vi "NewTemplate.GetBroadcasts.vi"(11 "NewTemplate in":refnum<class "Header.lvclass">) -> (2 "TemplateModule":cluster{"Broadcasts":T1, "Broadcasts":T2}, 3 "NewTemplate out":refnum<class "Header.lvclass">)   [LabVIEW 2024, in "Header.lvclass"]
uses:
  Header.lvclass
  JQMHCore/Module/StandardBroadcasts.ctl
  JQMHCore/Shared/Died.ctl
  JQMHCore/Module/Started.ctl
  Broadcast Events--cluster.ctl
  Stopped.ctl
  JQMHCore/Module/RQMHModule.lvclass/RQMHModule.ctl
  Header.lvclass/Header.ctl
  JQMHCore/Module/RQMHModule.lvclass
  C:/DevOps/CORTEX/JQMH/JQMHCore/Module/RQMHModule.lvclass
  C:/DevOps/CORTEX/JQMH/ModuleTemplates/Header/Header.lvclass
  JQMHCore/Shared/JQMHShared.lvlib
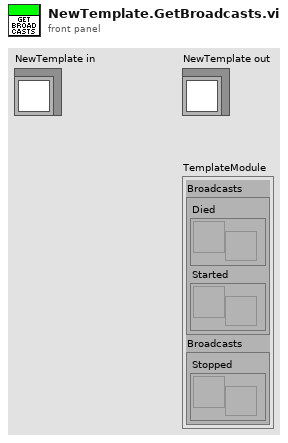
[diagram p1: front panel]
types:
  T1 = typedef "RQMHModule.lvclass/StandardBroadcasts.ctl" = cluster{"Died":refnum<user-event>, "Started":refnum<user-event>}
  T2 = typedef "Header.lvclass/Broadcast Events--cluster.ctl" = cluster{"Stopped":refnum<user-event>}
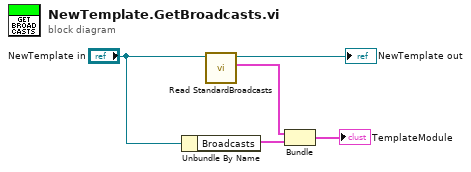
[diagram p0: block diagram]
diagram:
  n1 = Unbundle By Name("NewTemplate in") -> ("Broadcasts"=w5:T2)
  n2 = call "Read StandardBroadcasts.vi"("JQMHCore in"="NewTemplate in") -> ("Broadcasts"=w4:T1, "JQMHCore out"=→"NewTemplate out":refnum<class "Header.lvclass">)  [unwired: 8 in, 1 out]
  n3 = Bundle("Broadcasts"=w4, "Broadcasts"=w5) -> (→"TemplateModule":cluster{"Broadcasts":T1, "Broadcasts":T2})  [unwired: 1 in]
